vi "Write Data.vi"(8 "error in (no error)":errorcluster, 9 "Publication Time":timestamp, 10 "Value":variant, 11 "ValueReferenceTransport In":refnum<class "ValueReferenceTransport.lvclass">) -> (0 "error out":errorcluster, 3 "ValueReferenceTransport Out":refnum<class "ValueReferenceTransport.lvclass">)   [LabVIEW 2017, in "Transport.lvlib" / "ValueReferenceTransport.lvclass"]
doc: "<License>\nCopyright © 2017 Composed Systems, LLC | All rights reserved\nwww.composed.io\n\nAuthor: Ethan Stern <ethan.stern@composed.io>\n\nThis software is provided \"AS IS\" WITHOUT WARRANTIES, either express or implied, AND IS FOR EDUCATIONAL PURPOSES ONLY.\n</License>"
uses:
  ValueReferenceTransport.lvclass
  ValueReferenceTransport.lvclass/ValueReferenceTransport.ctl
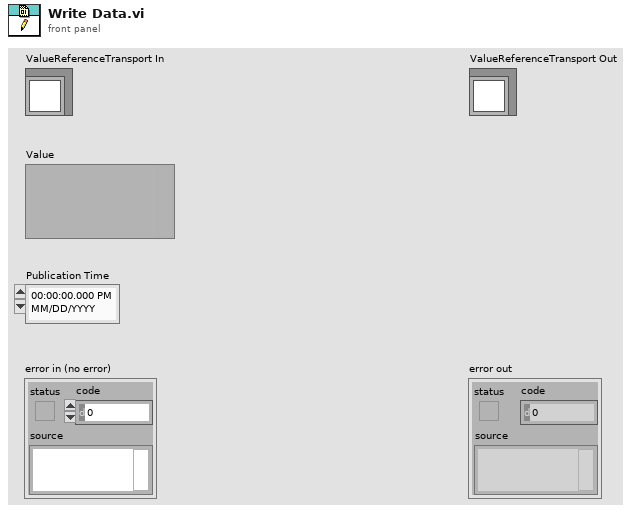
[diagram p1: front panel]
types:
  T1 = cluster{"Data":variant, "Publication Time":timestamp}
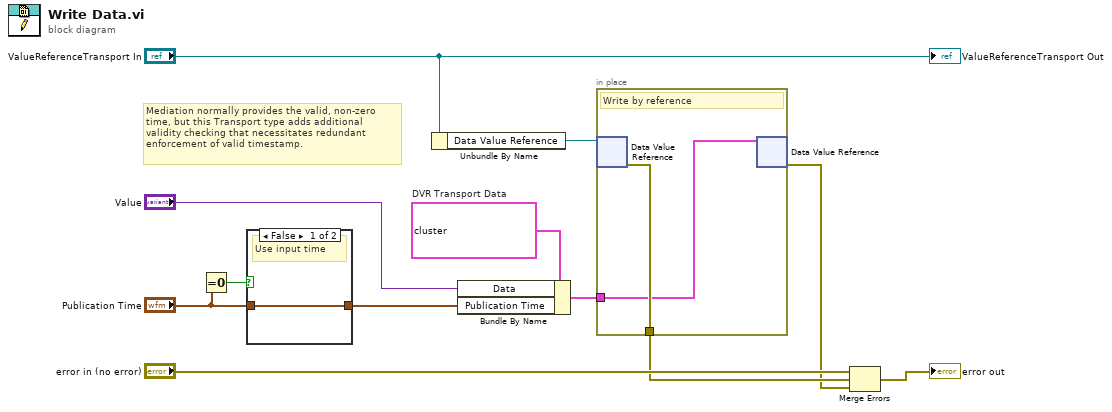
[diagram p0: block diagram]
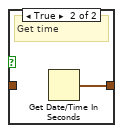
[diagram p2: hidden frame]
diagram:
  w6 = T1 {"Data"=variant, "Publication Time"=timestamp(0 s since 1904-01-01)}  # DVR Transport Data
  # "Mediation normally provides the valid, non-zero\ntime, but this Transport type adds additional\nvalidity checking that necessitates redundant\nenforcement of valid timestamp."
  n1 = Equal To 0?(x="Publication Time") -> (x = 0?=w3:bool)
  n2 = case shown="False" w3 {
    tunnel: "Publication Time" -> [w13 _]
    tunnel: [w13 w14] -> w1
    frame False {
      # "Use input time"
    }
    frame True {
      # "Get time"
      n3 = Get Date/Time In Seconds() -> (seconds since 1Jan1904=w14:timestamp)
    }
  }
  n4 = Unbundle By Name("ValueReferenceTransport In") -> ("Data Value Reference"=w9:refnum<data-value>)
  n5 = Bundle By Name(cluster=w6, "Data"="Value", "Publication Time"=w1) -> (w4:T1)
  n6 = in-place {
    in-place-border: [w16] -> w8
    in-place-border: w4 -> [w15]
    # "Write by reference"
    n7 = in-place-dvr #1(w9) -> (w16:errorcluster)  [unwired: 1 out]
    n8 = in-place-dvr #1(w15) -> (w7:errorcluster)  [unwired: 1 out]
  }
  n9 = Merge Errors("error in (no error)", w8, w7) -> (→"error out":errorcluster)
  "ValueReferenceTransport Out" <- "ValueReferenceTransport In"
